vi "AscriptPluginMain.vi"(9 "StopNotifier":refnum<notifier>, 10 "IPnotifier":refnum<notifier>, 11 "BasePath":path) -> ()   [LabVIEW 2016]
uses:
  <vilib>/Utility/file.llb/Read Delimited Spreadsheet (string).vi
  <vilib>/Rock Robotics/Network Tables/NT Write Boolean.vi
  <vilib>/FTP/NI_FTP.lvlib
panel:
  out "RobotIP":string
  in  "DeleteLog":bool
  in  "GetLogFile":bool
  out "Auto Script on Robot":string="GotThroughDef3noShoot"
  in  "DLfromRIO":bool
  in  "TemplateOpen":bool
  in  "Autoscript Layout":string(tree)
  in  "DeleteCommand":bool
  in  "SaveStep":bool
  in  "DeleteStep":bool
  in  "AddCmd":bool
  in  "Auto Script Name":string="GotThroughDef3noShoot"
  in  "AutoFiles":i32(listbox)=7
  in  "LoadAuto":bool
  in  "SaveAuto":bool
  in  "ULtoRIO":bool
  in  "ClearSteps":bool
  in  "AddStep":bool
  in  "DeleteAuto":bool
  in  "Return Variable Names":string[](array[string])
  in  "Arguments":string[](array[string])
  in  "Routine":string(combo)
  in  "LoadStep":bool
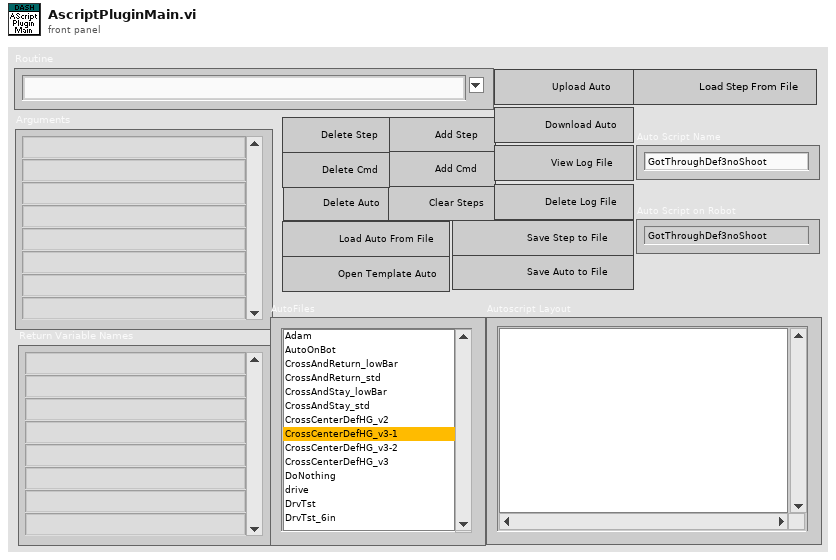
[diagram p1: front panel]
types:
  T1 = cluster{"Return Variable Names":refnum<vi>, "ArgumentsBox":refnum<vi>, "Routine":refnum<vi>, "AddCmd":refnum<vi>, "ClearSteps":refnum<vi>, "AddStep":refnum<vi>, "DeleteAuto":refnum<vi>, "DeleteCommand":refnum<vi>, "DeleteStep":refnum<vi>, "TemplateOpen":refnum<vi>, "SaveStep":refnum<vi>, "LoadAuto":refnum<vi>, "SaveAuto":refnum<vi>, "LoadStep":refnum<vi>, "AutoFiles":refnum<vi>, "DeleteLog":refnum<vi>, "GetLogFile":refnum<vi>, "Auto Script on Robot":refnum<vi>, "DLfromRIO":refnum<vi>, "Autoscript Layout":refnum<vi>, "Auto Script Name":refnum<vi>, "ULtoRIO":refnum<vi>}
  T2 = cluster{"Number":i32, "Name":string, "Commands":string[], "WaitForExecution":bool}
  T3 = enum16{"open", "replace", "create", "open or create", "replace or create", "replace or create with confirmation"}
  T4 = cluster{"Number":i32, "Name":string, "Commands":string[], "WaitForExecution":bool}[]
  T5 = typedef "NI_FTP.lvlib/FTP Session.ctl" = refnum<k5>
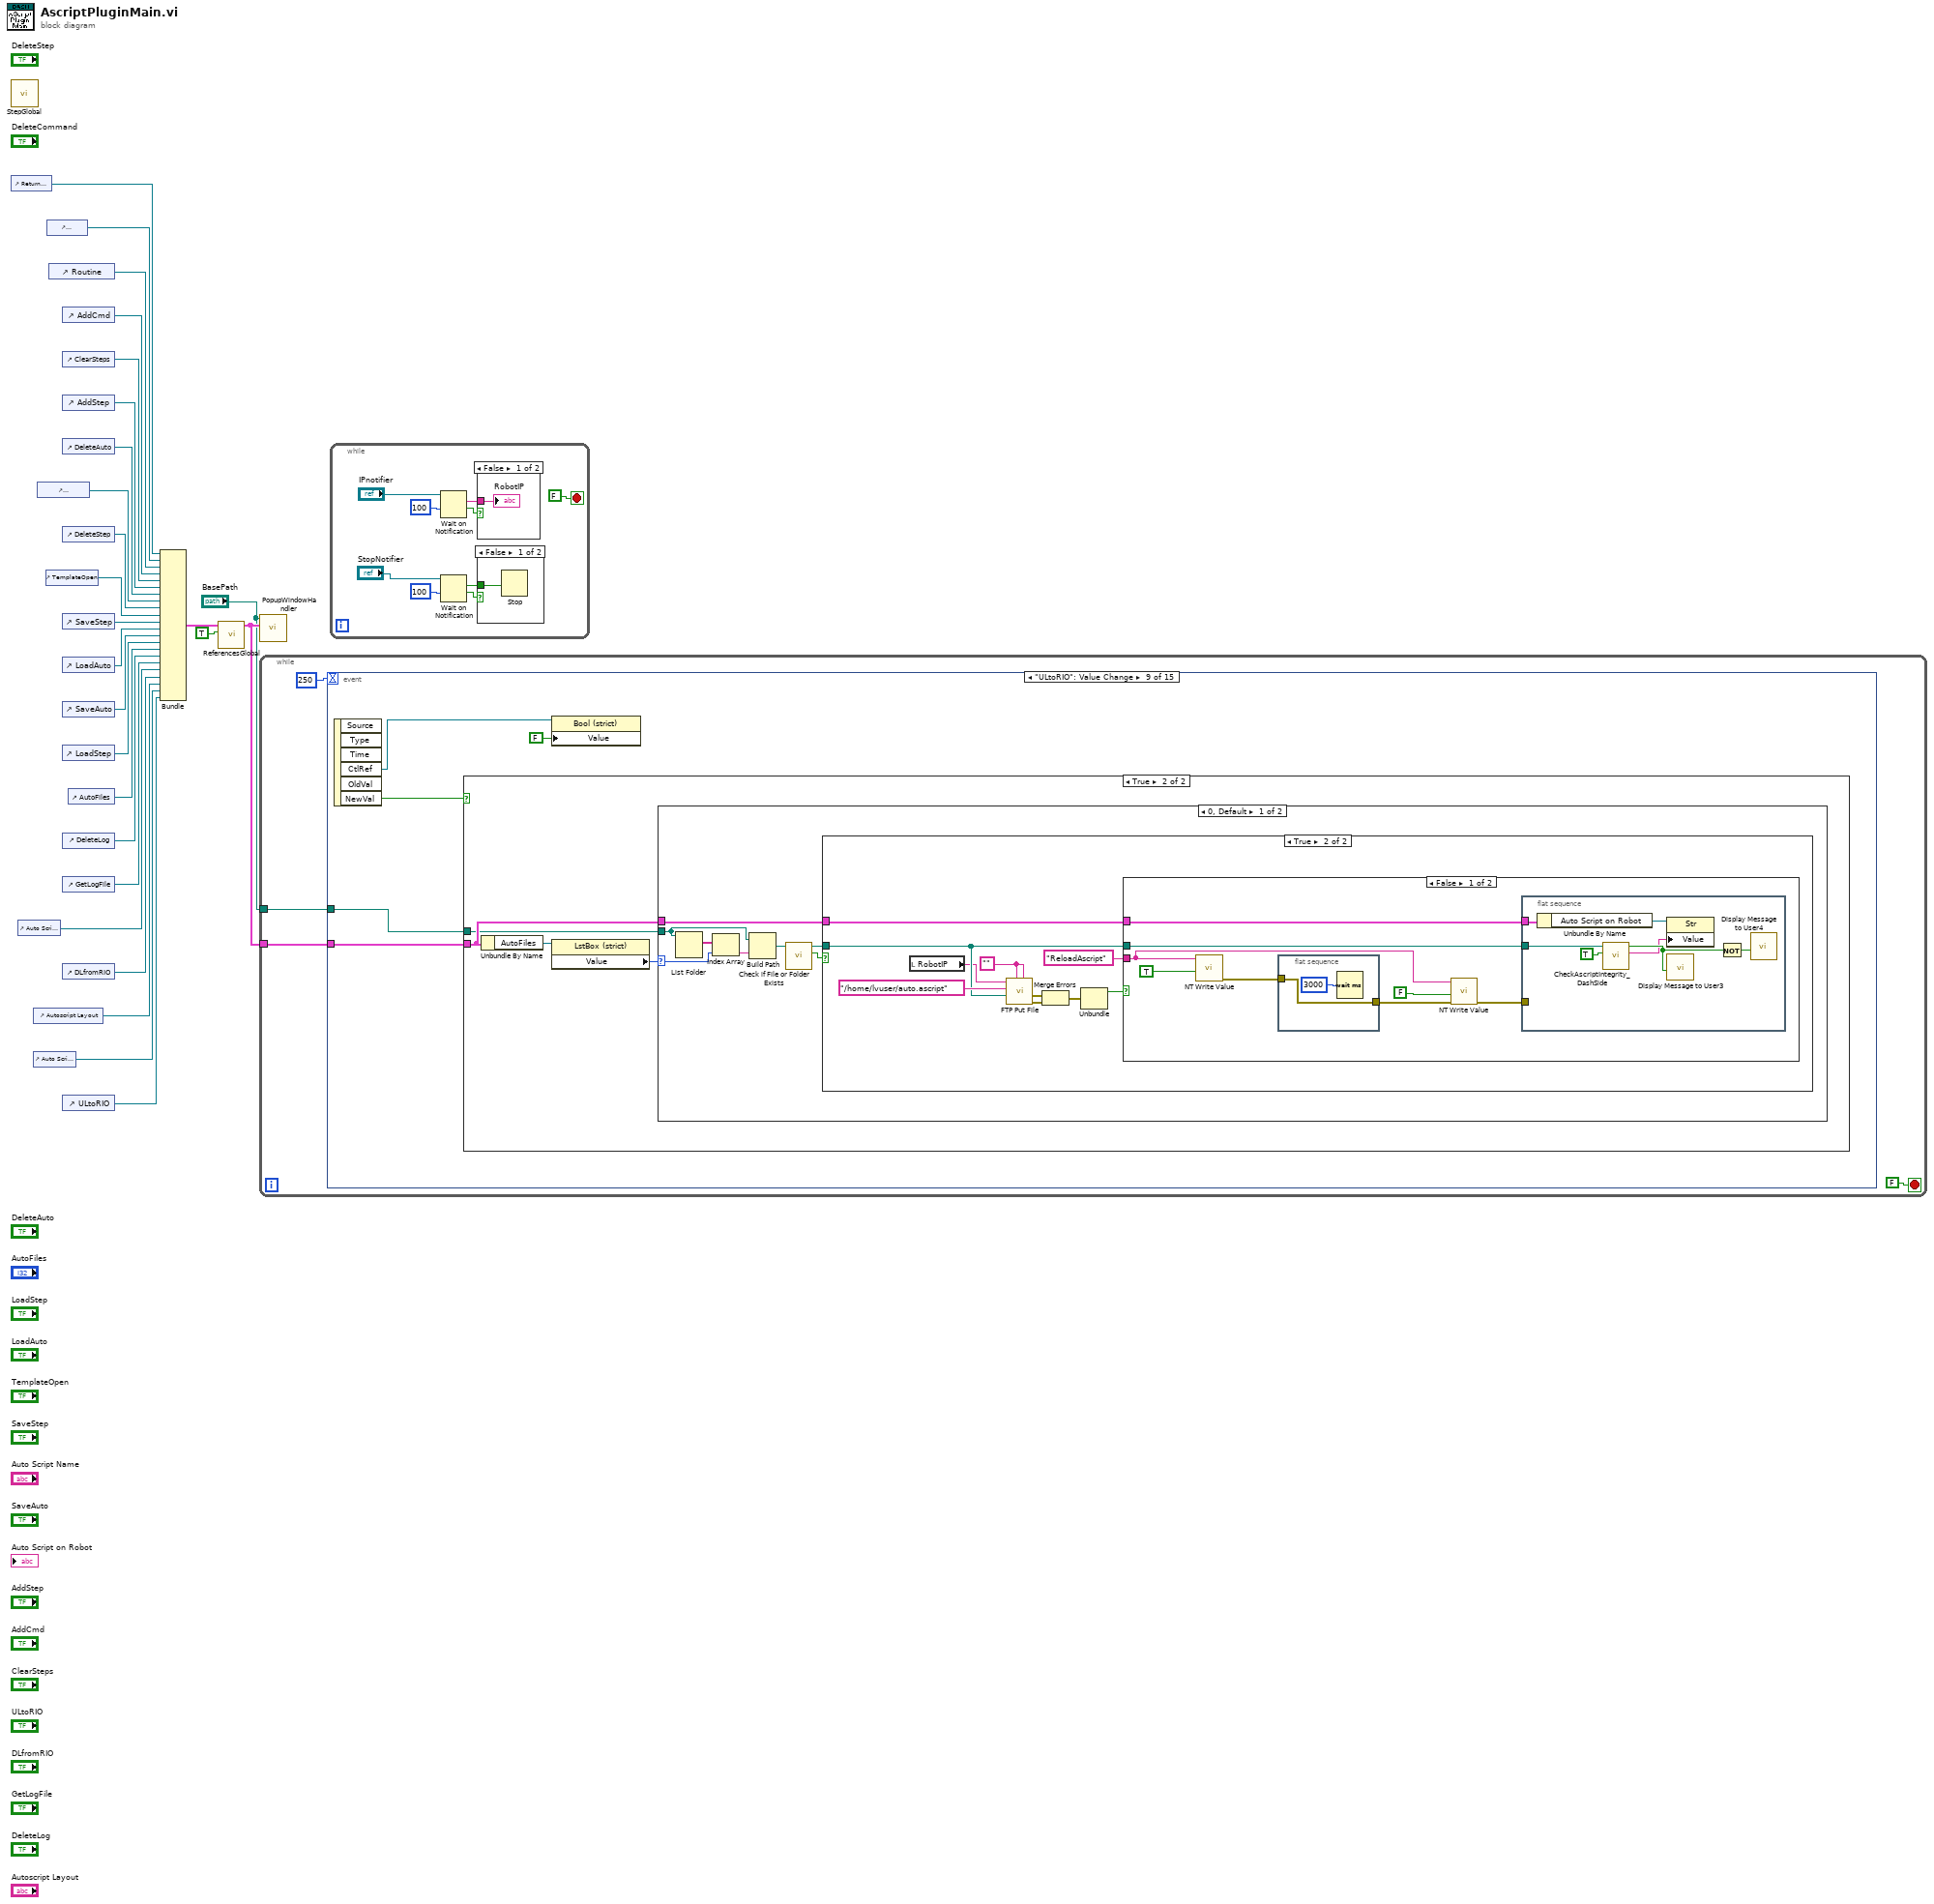
[diagram p0: block diagram]
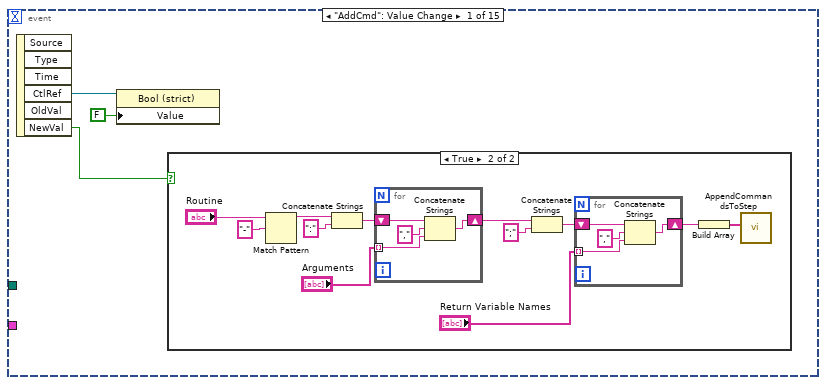
[diagram p2: hidden frame]
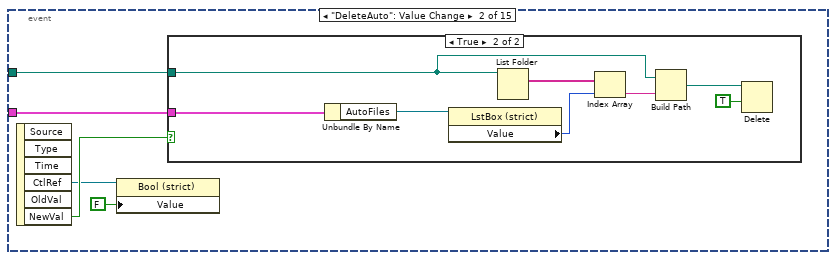
[diagram p4: hidden frame]
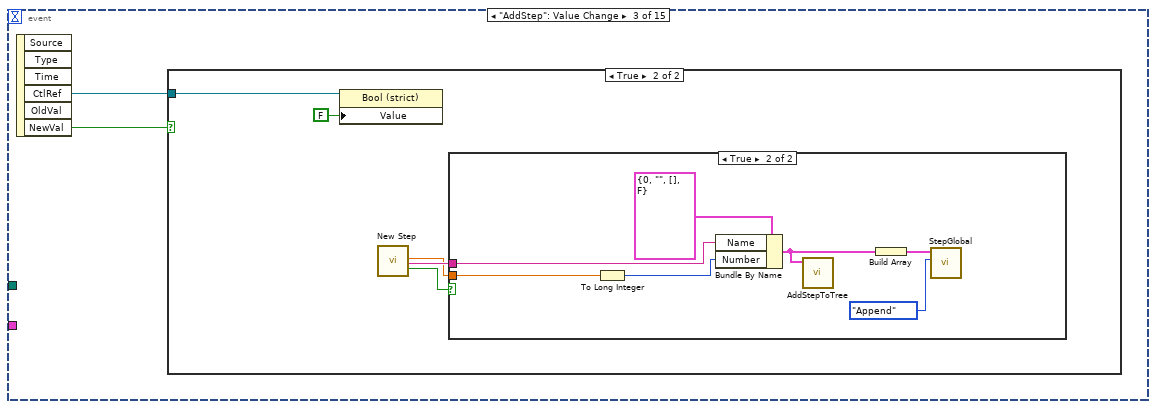
[diagram p6: hidden frame]
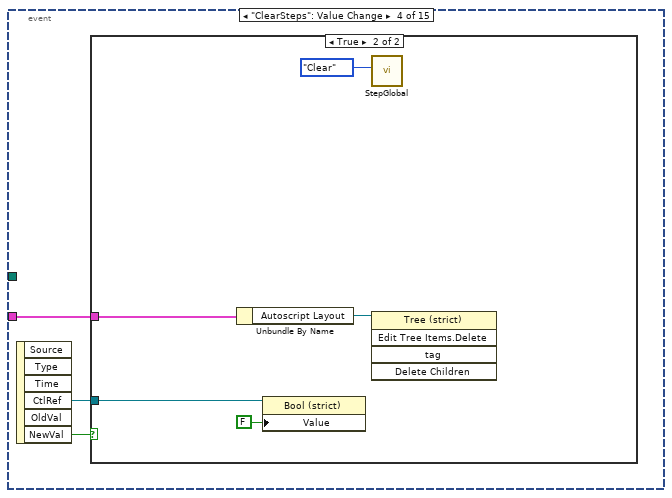
[diagram p9: hidden frame]
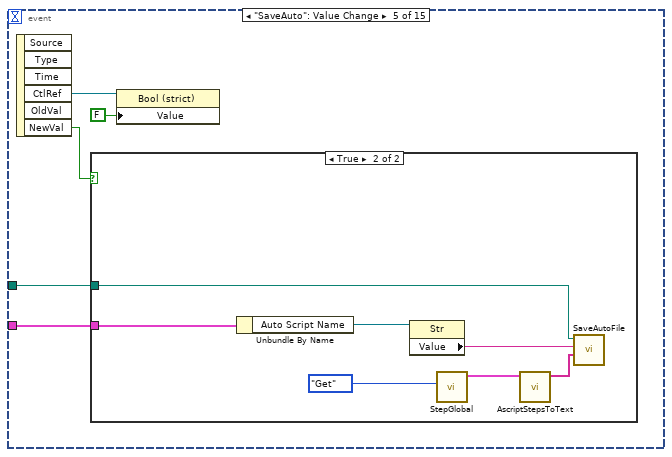
[diagram p11: hidden frame]
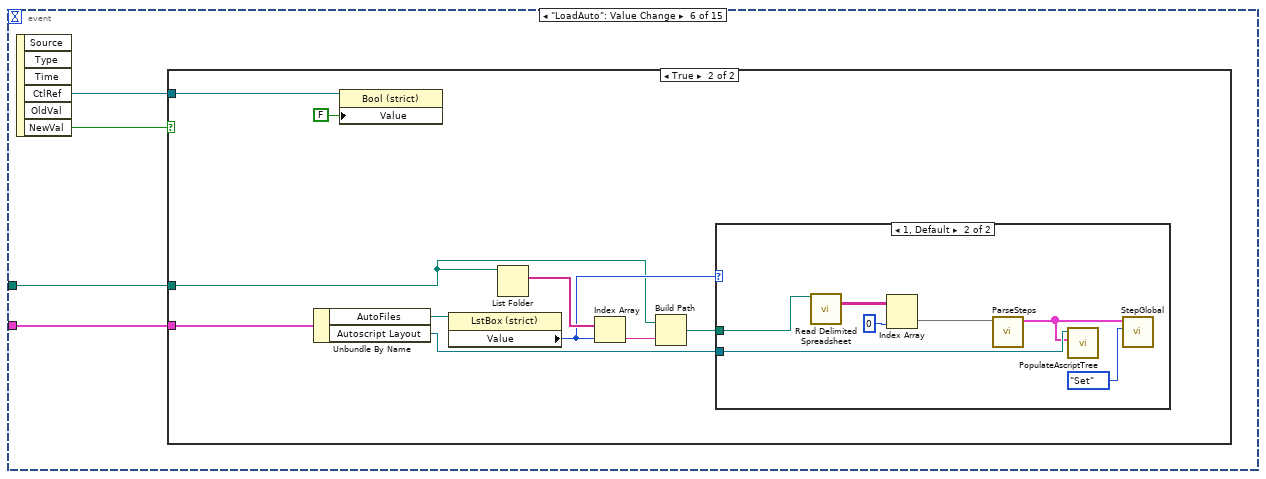
[diagram p13: hidden frame]
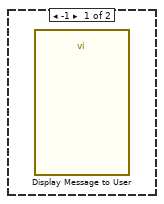
[diagram p15: hidden frame]
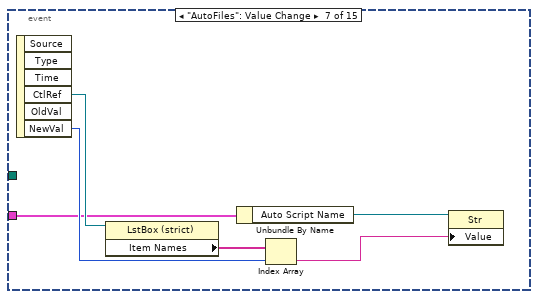
[diagram p16: hidden frame]
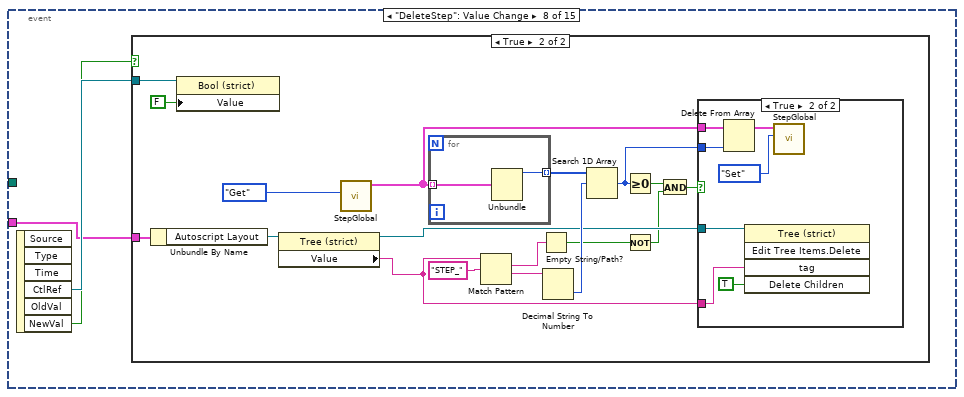
[diagram p17: hidden frame]
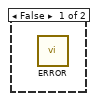
[diagram p19: hidden frame]
diagram:
  n1 = call "StepGlobal.vi"() -> ()  [unwired: 11 in, 1 out]
  n2 = control-ref of="Return Variable Names"() -> (w26:refnum<vi>)
  n3 = control-ref of="Auto Script on Robot"() -> (w9:refnum<vi>)
  n4 = control-ref of="Autoscript Layout"() -> (w7:refnum<vi>)
  n5 = control-ref of="Auto Script Name"() -> (w6:refnum<vi>)
  n6 = control-ref of="DeleteCommand"() -> (w19:refnum<vi>)
  n7 = control-ref of="TemplateOpen"() -> (w17:refnum<vi>)
  n8 = control-ref of="ArgumentsBox"() -> (w25:refnum<vi>)
  n9 = control-ref of="Routine"() -> (w24:refnum<vi>)
  n10 = control-ref of="AddCmd"() -> (w23:refnum<vi>)
  n11 = control-ref of="ClearSteps"() -> (w22:refnum<vi>)
  n12 = control-ref of="AddStep"() -> (w21:refnum<vi>)
  n13 = control-ref of="DeleteAuto"() -> (w20:refnum<vi>)
  n14 = control-ref of="DeleteStep"() -> (w18:refnum<vi>)
  n15 = control-ref of="SaveStep"() -> (w16:refnum<vi>)
  n16 = control-ref of="LoadAuto"() -> (w15:refnum<vi>)
  n17 = control-ref of="SaveAuto"() -> (w14:refnum<vi>)
  n18 = control-ref of="LoadStep"() -> (w13:refnum<vi>)
  n19 = control-ref of="DeleteLog"() -> (w10:refnum<vi>)
  n20 = control-ref of="GetLogFile"() -> (w11:refnum<vi>)
  n21 = control-ref of="DLfromRIO"() -> (w8:refnum<vi>)
  n22 = control-ref of="ULtoRIO"() -> (w5:refnum<vi>)
  n23 = control-ref of="AutoFiles"() -> (w12:refnum<vi>)
  n24 = Bundle("Return Variable Names"=w26, "ArgumentsBox"=w25, "Routine"=w24, "AddCmd"=w23, "ClearSteps"=w22, "AddStep"=w21, "DeleteAuto"=w20, "DeleteCommand"=w19, "DeleteStep"=w18, "TemplateOpen"=w17, "SaveStep"=w16, "LoadAuto"=w15, "SaveAuto"=w14, "LoadStep"=w13, "AutoFiles"=w12, "DeleteLog"=w10, "GetLogFile"=w11, "Auto Script on Robot"=w9, "DLfromRIO"=w8, "Autoscript Layout"=w7, "Auto Script Name"=w6, "ULtoRIO"=w5) -> (w4:T1)  [unwired: 1 in]
  n25 = call "ReferencesGlobal.vi"("Set?"=TRUE, "AscriptRefsIn"=w4) -> ("AscriptRefsOut"=w2:T1)  [unwired: 9 in]
  n26 = call "PopupWindowHandler.vi"("AscriptRefs"=w2, "BasePath"="BasePath") -> ()  [unwired: 10 in]
  n27 = while {
    tunnel: w2 -> [w30]
    tunnel: "BasePath" -> [w28]
    stop <- FALSE stop-if-true
    n28 = event shown="[8] \"ULtoRIO\": Value Change" {
      selector: _ -> [_ _ _ _ _ _ _ _ _ _ _ _ _ _ _]
      dyn-events: _ -> [_ _ _ _ _ _ _ _ _ _ _ _ _ _ _]
      timeout: 250 -> [_ _ _ _ _ _ _ _ _ _ _ _ _ _ _]
      tunnel: w30 -> [_ w58 _ w81 w93 w101 w122 w128 w162 _ w229 w262 _ _ w370]
      tunnel: w28 -> [_ w56 _ _ w92 w104 _ _ w161 w202 _ w258 w288 _ w369]
      event "AddCmd": Value Change {
        n29 = event-data() -> ("CtlRef"=w32:refnum<vi>, "NewVal"=w33:bool)  [unwired: 1 in, 4 out]
        n30 = property class="Bool (strict)"(reference=w32, "Value"=FALSE) -> ()  [unwired: 1 in, 2 out]
        n31 = case shown="True" w33 {
          frame False {
          }
          frame True {
            n32 = Match Pattern(string="Routine", regular expression="-") -> (before substring=w40:string)  [unwired: 1 in, 3 out]
            n33 = Concatenate Strings(w40, ":" ("string")) -> (w43:string)
            n34 = for {
              tunnel: "Arguments" -> [w52] mode=indexing
              shift-right: [w50] -> w35
              shift-left: w43 -> [w51]
              n35 = Concatenate Strings(w51, "," ("string"), w52) -> (w50:string)
            }
            n36 = Concatenate Strings(w35, ";" ("string")) -> (w37:string)
            n37 = for {
              tunnel: "Return Variable Names" -> [w48] mode=indexing
              shift-right: [w46] -> w34
              shift-left: w37 -> [w47]
              n38 = Concatenate Strings(w47, "," ("string"), w48) -> (w46:string)
            }
            n39 = Build Array(w34) -> (w45:string[])
            n40 = call "AppendCommandsToStep.vi"("CommandsToAppend"=w45) -> ()  [unwired: 11 in]
          }
        }
      }
      event "DeleteAuto": Value Change {
        n41 = event-data() -> ("CtlRef"=w54:refnum<vi>, "NewVal"=w57:bool)  [unwired: 1 in, 4 out]
        n42 = property class="Bool (strict)"(reference=w54, "Value"=FALSE) -> ()  [unwired: 1 in, 2 out]
        n43 = case shown="True" w57 {
          tunnel: w58 -> [_ w66]
          tunnel: w56 -> [_ w59]
          frame False {
          }
          frame True {
            n44 = Unbundle By Name(w66) -> ("AutoFiles"=w65:refnum<vi>)
            n45 = property class="LstBox (strict)"(reference=w65) -> ("Value"=w63:i32)  [unwired: 1 in, 2 out]
            n46 = List Folder(path=w59) -> (filenames=w64:string[])  [unwired: 3 in, 3 out]
            n47 = Index Array(array=w64, index=w63) -> (element=w62:string)
            n48 = Build Path(base path=w59, name or relative path=w62) -> (appended path=w60:path)
            n49 = Delete(path (use dialog)=w60, confirm (F)=TRUE) -> ()  [unwired: 3 in, 3 out]
          }
        }
      }
      event "AddStep": Value Change {
        n50 = event-data() -> ("CtlRef"=w68:refnum<vi>, "NewVal"=w67:bool)  [unwired: 1 in, 4 out]
        n51 = case shown="True" w67 {
          tunnel: w68 -> [_ w73]
          frame False {
          }
          frame True {
            n52 = property class="Bool (strict)"(reference=w73, "Value"=FALSE) -> ()  [unwired: 1 in, 2 out]
            n53 = call "New Step"() -> ("Step Number"=w69:dbl, "Step Name"=w70:string, "OK"=w71:bool)  [unwired: 16 in, 1 out]
            n54 = case shown="True" w71 {
              tunnel: w70 -> [_ w77]
              tunnel: w69 -> [_ w80]
              frame False {
              }
              frame True {
                n55 = To Long Integer(number=w80) -> (32bit integer=w78:i32)
                n56 = Bundle By Name(cluster=T2 {"Number"=0, "Name"="", "Commands"=[], "WaitForExecution"=FALSE} ("Step"), "Name"=w77, "Number"=w78) -> (w76:T2)
                n57 = call "AddStepToTree.vi"("Step"=w76) -> ()  [unwired: 10 in, 1 out]
                n58 = Build Array(w76) -> (w75:T4)
                n59 = call "StepGlobal.vi"("Action (Get)"=enum16{"Clear", "Append", "Set", "Get"}."Append" ("Action"), "AutoScriptSteps in"=w75) -> ()  [unwired: 9 in, 1 out]
              }
            }
          }
        }
      }
      event "ClearSteps": Value Change {
        n60 = event-data() -> ("CtlRef"=w83:refnum<vi>, "NewVal"=w82:bool)  [unwired: 1 in, 4 out]
        n61 = case shown="True" w82 {
          tunnel: w83 -> [_ w87]
          tunnel: w81 -> [_ w86]
          frame False {
          }
          frame True {
            n62 = Unbundle By Name(w86) -> ("Autoscript Layout"=w85:refnum<vi>)
            n63 = property class="Bool (strict)"(reference=w87, "Value"=FALSE) -> ()  [unwired: 1 in, 2 out]
            n64 = call "StepGlobal.vi"("Action (Get)"=enum16{"Clear", "Append", "Set", "Get"}."Clear" ("Action")) -> ()  [unwired: 10 in, 1 out]
            n65 = invoke class="Tree (strict)" method="Edit Tree Items.Delete"(reference=w85) -> ()  [unwired: 4 in, 5 out]
          }
        }
      }
      event "SaveAuto": Value Change {
        n66 = event-data() -> ("CtlRef"=w89:refnum<vi>, "NewVal"=w91:bool)  [unwired: 1 in, 4 out]
        n67 = case shown="True" w91 {
          tunnel: w93 -> [_ w100]
          tunnel: w92 -> [_ w94]
          frame False {
          }
          frame True {
            n68 = Unbundle By Name(w100) -> ("Auto Script Name"=w99:refnum<vi>)
            n69 = property class="Str"(reference=w99) -> ("Value"=w98:string)  [unwired: 1 in, 2 out]
            n70 = call "StepGlobal.vi"("Action (Get)"=enum16{"Clear", "Append", "Set", "Get"}."Get" ("Action")) -> ("AutoScriptSteps out"=w96:T4)  [unwired: 10 in]
            n71 = call "AscriptStepsToText.vi"("AutoScriptSteps"=w96) -> ("AscriptLines"=w97:string[])  [unwired: 10 in]
            n72 = call "SaveAutoFile.vi"("Ascript Data"=w97, "Filename"=w98, "Base path"=w94) -> ()  [unwired: 8 in, 1 out]
          }
        }
        n73 = property class="Bool (strict)"(reference=w89, "Value"=FALSE) -> ()  [unwired: 1 in, 2 out]
      }
      event "LoadAuto": Value Change {
        n74 = event-data() -> ("CtlRef"=w103:refnum<vi>, "NewVal"=w102:bool)  [unwired: 1 in, 4 out]
        n75 = case shown="True" w102 {
          tunnel: w101 -> [_ w110]
          tunnel: w103 -> [_ w109]
          tunnel: w104 -> [_ w105]
          frame False {
          }
          frame True {
            n76 = Unbundle By Name(w110) -> ("AutoFiles"=w113:refnum<vi>, "Autoscript Layout"=w106:refnum<vi>)
            n77 = property class="Bool (strict)"(reference=w109, "Value"=FALSE ("Panel Transparent")) -> ()  [unwired: 1 in, 2 out]
            n78 = property class="LstBox (strict)"(reference=w113) -> ("Value"=w108:i32)  [unwired: 1 in, 2 out]
            n79 = List Folder(path=w105) -> (filenames=w112:string[])  [unwired: 3 in, 3 out]
            n80 = Index Array(array=w112, index=w108) -> (element=w111:string)
            n81 = Build Path(base path=w105, name or relative path=w111) -> (appended path=w107:path)
            n82 = case shown="1, Default" w108 {
              tunnel: w107 -> [_ w121]
              tunnel: w106 -> [_ w117]
              frame -1 {
                n83 = call "Display Message to User"() -> ()  [unwired: 10 in, 2 out]
              }
              frame 1, Default {
                n84 = call-poly <vilib>:"Read Delimited Spreadsheet.vi"("file path (dialog if empty)"=w121) -> ("all rows"=w120:string[][])  [unwired: 9 in, 5 out]
                n85 = Index Array(array=w120, index (col)=0 ("disabled index (col)")) -> (element=w118:string[])  [unwired: 1 in]
                n86 = call "ParseSteps.vi"("AscriptLines"=w118) -> ("Steps"=w116:T4)  [unwired: 10 in]
                n87 = call "PopulateAscriptTree.vi"("Steps in"=w116, "Autoscript Layout"=w117) -> ()  [unwired: 8 in, 2 out]
                n88 = call "StepGlobal.vi"("Action (Get)"=enum16{"Clear", "Append", "Set", "Get"}."Set" ("Action"), "AutoScriptSteps in"=w116) -> ()  [unwired: 9 in, 1 out]
              }
            }
          }
        }
      }
      event "AutoFiles": Value Change {
        n89 = event-data() -> ("CtlRef"=w124:refnum<vi>, "NewVal"=w123:i32)  [unwired: 1 in, 4 out]
        n90 = property class="LstBox (strict)"(reference=w124) -> ("Item Names"=w125:string[])  [unwired: 1 in, 2 out]
        n91 = Unbundle By Name(w122) -> ("Auto Script Name"=w126:refnum<vi>)
        n92 = Index Array(array=w125, index=w123) -> (element=w127:string)
        n93 = property class="Str"(reference=w126, "Value"=w127) -> ()  [unwired: 1 in, 2 out]
      }
      event "DeleteStep": Value Change {
        n94 = event-data() -> ("CtlRef"=w130:refnum<vi>, "NewVal"=w129:bool)  [unwired: 1 in, 4 out]
        n95 = case shown="True" w129 {
          tunnel: w130 -> [_ w147]
          tunnel: w128 -> [_ w141]
          frame False {
          }
          frame True {
            n96 = Unbundle By Name(w141) -> ("Autoscript Layout"=w140:refnum<vi>)
            n97 = property class="Bool (strict)"(reference=w147, "Value"=FALSE ("Panel Transparent")) -> ()  [unwired: 1 in, 2 out]
            n98 = property class="Tree (strict)"(reference=w140) -> (reference out=w136:refnum<vi>, "Value"=w131:string)  [unwired: 1 in, 1 out]
            n99 = call "StepGlobal.vi"("Action (Get)"=enum16{"Clear", "Append", "Set", "Get"}."Get" ("Action")) -> ("AutoScriptSteps out"=w133:T4)  [unwired: 10 in]
            n100 = for {
              tunnel: w133 -> [w157] mode=indexing
              tunnel: [w156] -> w143 mode=indexing
              n101 = Unbundle(w157) -> ("Number"=w156:i32)  [unwired: 3 out]
            }
            n102 = Match Pattern(string=w131, regular expression="STEP_") -> (match substring=w137:string, after substring=w145:string)  [unwired: 1 in, 2 out]
            n103 = Empty String/Path?(string/path=w137) -> (empty?=w135:bool)
            n104 = Decimal String To Number(string=w145) -> (number=w144:i32)  [unwired: 2 in, 1 out]
            n105 = Search 1D Array(1D array=w143, element=w144) -> (index of element=w142:i32)  [unwired: 1 in]
            n106 = Greater Or Equal To 0?(x=w142) -> (x >= 0?=w139:bool)
            n107 = Not(x=w135) -> (.not. x?=w134:bool)
            n108 = And(x=w139, y=w134) -> (x .and. y?=w138:bool)
            n109 = case shown="True" w138 {
              tunnel: w142 -> [_ w155]
              tunnel: w133 -> [_ w154]
              tunnel: w136 -> [_ w153]
              tunnel: w131 -> [_ w152]
              frame False {
                n110 = call "ERROR"() -> ()  [unwired: 10 in, 2 out]
              }
              frame True {
                n111 = Delete From Array(array=w154, index=w155) -> (array with subset deleted=w150:T4)  [unwired: 1 in, 1 out]
                n112 = invoke class="Tree (strict)" method="Edit Tree Items.Delete"(reference=w153, "tag"=w152, "Delete Children"=TRUE ("Delete Children?")) -> ()  [unwired: 2 in, 5 out]
                n113 = call "StepGlobal.vi"("Action (Get)"=enum16{"Clear", "Append", "Set", "Get"}."Set" ("Action"), "AutoScriptSteps in"=w150) -> ()  [unwired: 9 in, 1 out]
              }
            }
          }
        }
      }
      event "ULtoRIO": Value Change {
        n114 = event-data() -> ("CtlRef"=w158:refnum<vi>, "NewVal"=w160:bool)  [unwired: 1 in, 4 out]
        n115 = case shown="True" w160 {
          tunnel: w162 -> [_ w164]
          tunnel: w161 -> [_ w163]
          frame False {
          }
          frame True {
            n116 = Unbundle By Name(w164) -> ("AutoFiles"=w166:refnum<vi>)
            n117 = property class="LstBox (strict)"(reference=w166) -> ("Value"=w165:i32)  [unwired: 1 in, 2 out]
            n118 = case shown="0, Default" w165 {
              selector: w165 -> [w172 _]
              tunnel: w164 -> [w168 _]
              tunnel: w163 -> [w167 _]
              frame 0, Default {
                n119 = List Folder(path=w167) -> (filenames=w174:string[])  [unwired: 3 in, 3 out]
                n120 = Index Array(array=w174, index=w172) -> (element=w173:string)
                n121 = Build Path(base path=w167, name or relative path=w173) -> (appended path=w171:path)
                n122 = call <vilib>:"Check if File or Folder Exists.vi"("path"=w171) -> ("file or folder exists?"=w170:bool, "dup path"=w169:path)  [unwired: 8 in, 1 out]
                n123 = case shown="True" w170 {
                  tunnel: w169 -> [_ w177]
                  tunnel: w168 -> [_ w176]
                  frame False {
                    n124 = call "Display Message to User2"() -> ()  [unwired: 10 in, 2 out]
                  }
                  frame True {
                    w180 = ""
                    n125 = local read "RobotIP"() -> (w175:string)
                    n126 = call <vilib>:"FTP Put File.vi"("password"=w180, "user"=w180, "local path"=w177, "remote path"="/home/lvuser/auto.ascript" ("remote path (roboRIO)"), "host"=w175) -> ("error out"=w183:errorcluster, "file error"=w184:errorcluster)  [unwired: 5 in]
                    n127 = Merge Errors(w184, w183) -> (w182:errorcluster)
                    n128 = Unbundle(w182) -> ("status"=w179:bool)  [unwired: 2 out]
                    n129 = case shown="False" w179 {
                      tunnel: "ReloadAscript" ("remote path (roboRIO)") -> [w189 _]
                      tunnel: w177 -> [w186 _]
                      tunnel: w176 -> [w185 _]
                      frame False {
                        n130 = call-poly <vilib>:"NT Write Value.vi"("Boolean"=TRUE, "Name"=w189) -> ("error out"=w191:errorcluster)  [unwired: 9 in]
                        n131 = flat-sequence {
                          tunnel: w191 -> [w200]
                          tunnel: [w200] -> w190
                          frame #0 {
                            n132 = Wait (ms)(milliseconds to wait=u32 3000) -> ()  [unwired: 1 out]
                          }
                        }
                        n133 = call-poly <vilib>:"NT Write Value.vi"("error in"=w190, "Boolean"=FALSE, "Name"=w189) -> ("error out"=w187:errorcluster)  [unwired: 8 in]
                        n134 = flat-sequence {
                          tunnel: w187 -> [_]
                          tunnel: w186 -> [w198]
                          tunnel: w185 -> [w195]
                          frame #0 {
                            n135 = Unbundle By Name(w195) -> ("Auto Script on Robot"=w194:refnum<vi>)
                            n136 = call "CheckAscriptIntegrity_DashSide.vi"("UseUploadedPath?"=TRUE, "UploadedAscript"=w198) -> ("BotAscriptName"=w193:string, "AscriptIntegrityGood?"=w196:bool)  [unwired: 8 in]
                            n137 = property class="Str"(reference=w194, "Value"=w193) -> ()  [unwired: 1 in, 2 out]
                            n138 = call "Display Message to User3"("Enable"=w196) -> ()  [unwired: 9 in, 2 out]
                            n139 = Not(x=w196) -> (.not. x?=w197:bool)
                            n140 = call "Display Message to User4"("Enable"=w197) -> ()  [unwired: 9 in, 2 out]
                          }
                        }
                      }
                      frame True {
                        n141 = call "Display Message to User5"() -> ()  [unwired: 10 in, 2 out]
                      }
                    }
                  }
                }
              }
              frame -1 {
                n142 = call "Display Message to User6"() -> ()  [unwired: 10 in, 2 out]
              }
            }
          }
        }
        n143 = property class="Bool (strict)"(reference=w158, "Value"=FALSE ("Panel Transparent")) -> ()  [unwired: 1 in, 2 out]
      }
      event "SaveStep": Value Change {
        n144 = event-data() -> ("CtlRef"=w203:refnum<vi>, "NewVal"=w204:bool)  [unwired: 1 in, 4 out]
        n145 = case shown="True" w204 {
          tunnel: w203 -> [_ w206]
          tunnel: w202 -> [_ w205]
          frame False {
          }
          frame True {
            n146 = property class="Bool (strict)"(reference=w206, "Value"=FALSE) -> ()  [unwired: 1 in, 2 out]
            n147 = call "Save Step"() -> ("Step Name"=w207:string, "Use Existing Step Name?"=w208:bool, "Step Number"=w210:dbl, "OK"=w211:bool)  [unwired: 15 in, 1 out]
            n148 = To Long Integer(number=w210) -> (32bit integer=w209:i32)
            n149 = case shown="True" w211 {
              tunnel: w209 -> [_ w220]
              tunnel: w208 -> [_ w218]
              tunnel: w207 -> [_ w216]
              tunnel: w205 -> [_ w213]
              frame False {
              }
              frame True {
                n150 = call "StepGlobal.vi"() -> ("AutoScriptSteps out"=w214:T4)  [unwired: 11 in]
                n151 = for {
                  tunnel: w214 -> [w227] mode=indexing
                  tunnel: [w226] -> w221 mode=indexing
                  n152 = Unbundle(w227) -> ("Number"=w226:i32)  [unwired: 3 out]
                }
                n153 = Search 1D Array(1D array=w221, element=w220) -> (index of element=w219:i32)  [unwired: 1 in]
                n154 = Index Array(array=w214, index=w219) -> (element=w217:T2)
                n155 = case shown="True" w218 {
                  tunnel: w217 -> [w224 w225]
                  tunnel: w216 -> [w223 _]
                  tunnel: [w222 w225] -> w215
                  frame False {
                    n156 = Bundle By Name(cluster=w224, "Name"=w223) -> (w222:T2)
                  }
                  frame True {
                  }
                }
                n157 = call "SaveStepToFile.vi"("base path"=w213, "Step"=w215) -> ()  [unwired: 10 in]
              }
            }
          }
        }
      }
      event "DeleteCommand": Value Change {
        n158 = event-data() -> ("CtlRef"=w230:refnum<vi>, "NewVal"=w228:bool)  [unwired: 1 in, 4 out]
        n159 = property class="Bool (strict)"(reference=w230, "Value"=FALSE) -> ()  [unwired: 1 in, 2 out]
        n160 = case shown="True" w228 {
          tunnel: w229 -> [_ w236]
          frame False {
          }
          frame True {
            n161 = Unbundle By Name(w236) -> ("Autoscript Layout"=w235:refnum<vi>)
            n162 = property class="Tree (strict)"(reference=w235) -> (reference out=w233:refnum<vi>, "Value"=w232:string)  [unwired: 1 in, 1 out]
            n163 = Empty String/Path?(string/path=w232) -> (empty?=w234:bool)
            n164 = case shown="False" w234 {
              tunnel: w232 -> [w241 _]
              tunnel: w233 -> [w240 _]
              frame False {
                n165 = invoke class="Tree (strict)" method="Edit Tree Items.Delete"(reference=w240, "tag"=w241, "Delete Children"=TRUE ("Delete Children?")) -> ()  [unwired: 2 in, 5 out]
                n166 = call "StepGlobal.vi"() -> ("AutoScriptSteps out"=w239:T4)  [unwired: 11 in]
                n167 = Match Pattern(string=w241, regular expression="_") -> (before substring=w245:string, after substring=w246:string)  [unwired: 1 in, 2 out]
                n168 = for {
                  tunnel: w239 -> [w257] mode=indexing
                  tunnel: [w256] -> w249 mode=indexing
                  n169 = Unbundle By Name(w257) -> ("Number"=w256:i32)
                }
                n170 = Decimal String To Number(string=w245) -> (number=w244:i32)  [unwired: 2 in, 1 out]
                n171 = Decimal String To Number(string=w246) -> (number=w243:i32)  [unwired: 2 in, 1 out]
                n172 = Search 1D Array(1D array=w249, element=w244) -> (index of element=w248:i32)  [unwired: 1 in]
                n173 = in-place {
                  in-place-border: w243 -> [w251]
                  n174 = in-place-array #1(w239, w248) -> (w252:T2)
                  n175 = in-place {
                    in-place-border: w251 -> [w253]
                    n176 = in-place-cluster #2(w252) -> ("Commands"=w255:string[])
                    n177 = Delete From Array(array=w255, index=w253) -> (array with subset deleted=w254:string[])  [unwired: 1 in, 1 out]
                    n178 = in-place-cluster #2("Commands"=w254) -> (w250:T2)
                  }
                  n179 = in-place-array #1(w250) -> (w238:T4)  [unwired: 1 out]
                }
                n180 = call "StepGlobal.vi"("Action (Get)"=enum16{"Clear", "Append", "Set", "Get"}."Set", "AutoScriptSteps in"=w238) -> ()  [unwired: 9 in, 1 out]
              }
              frame True {
              }
            }
          }
        }
      }
      event "DLfromRIO": Value Change {
        n181 = event-data() -> ("CtlRef"=w259:refnum<vi>, "NewVal"=w261:bool)  [unwired: 1 in, 4 out]
        n182 = property class="Bool (strict)"(reference=w259, "Value"=FALSE) -> ()  [unwired: 1 in, 2 out]
        n183 = case shown="True" w261 {
          tunnel: w262 -> [_ w266]
          tunnel: w258 -> [_ w264]
          frame False {
          }
          frame True {
            w275 = ""
            n184 = call <vilib>:"Check if File or Folder Exists.vi"("path"=w264) -> ("file or folder exists?"=w277:bool, "dup path"=w276:path)  [unwired: 8 in, 1 out]
            n185 = case shown="False" w277 {
              tunnel: w276 -> [w286 w287]
              tunnel: [w285 w287] -> w273
              frame False {
                n186 = Create Folder(path (use dialog)=w286) -> (created path=w285:path)  [unwired: 2 in, 2 out]
              }
              frame True {
              }
            }
            n187 = local read "RobotIP"() -> (w263:string)
            n188 = Build Path(base path=w273, name or relative path="AutoOnBot.ascript") -> (appended path=w267:path)
            n189 = call <vilib>:"FTP Get File.vi"("password"=w275, "user"=w275, "local path"=w267, "remote path"="/home/lvuser/auto.ascript", "host"=w263) -> ("error out"=w270:errorcluster, "file error"=w271:errorcluster)  [unwired: 5 in]
            n190 = Unbundle By Name(w266) -> ("Autoscript Layout"=w265:refnum<vi>)
            n191 = Merge Errors(w271, w270) -> (w269:errorcluster)
            n192 = Unbundle(w269) -> ("status"=w268:bool)  [unwired: 2 out]
            n193 = case shown="False" w268 {
              tunnel: w267 -> [w281 _]
              tunnel: w265 -> [w280 _]
              frame False {
                n194 = call-poly <vilib>:"Read Delimited Spreadsheet.vi"("file path (dialog if empty)"=w281) -> ("all rows"=w284:string[][])  [unwired: 9 in, 5 out]
                n195 = Index Array(array=w284, index (col)=0 ("disabled index (col)")) -> (element=w282:string[])  [unwired: 1 in]
                n196 = call "ParseSteps.vi"("AscriptLines"=w282) -> ("Steps"=w279:T4)  [unwired: 10 in]
                n197 = call "PopulateAscriptTree.vi"("Steps in"=w279, "Autoscript Layout"=w280) -> ()  [unwired: 8 in, 2 out]
                n198 = call "StepGlobal.vi"("Action (Get)"=enum16{"Clear", "Append", "Set", "Get"}."Set", "AutoScriptSteps in"=w279) -> ()  [unwired: 9 in, 1 out]
              }
              frame True {
                n199 = call "Display Message to User7"() -> ()  [unwired: 10 in, 2 out]
              }
            }
          }
        }
      }
      event "GetLogFile": Value Change {
        n200 = event-data() -> ("CtlRef"=w289:refnum<vi>, "NewVal"=w290:bool)  [unwired: 1 in, 4 out]
        n201 = property class="Bool (strict)"(reference=w289, "Value"=FALSE) -> ()  [unwired: 1 in, 2 out]
        n202 = case shown="True" w290 {
          tunnel: w288 -> [_ w293]
          frame False {
          }
          frame True {
            w304 = ""
            n203 = Build Path(base path=w293, name or relative path="AutoLogFiles") -> (appended path=w307:path)
            n204 = call <vilib>:"Check if File or Folder Exists.vi"("path"=w307) -> ("file or folder exists?"=w306:bool, "dup path"=w305:path)  [unwired: 8 in, 1 out]
            n205 = case shown="False" w306 {
              tunnel: w305 -> [w316 w317]
              tunnel: [w315 w317] -> w302
              frame False {
                n206 = Create Folder(path (use dialog)=w316) -> (created path=w315:path)  [unwired: 2 in, 2 out]
              }
              frame True {
              }
            }
            n207 = Get Date/Time In Seconds() -> (seconds since 1Jan1904=w298:timestamp)
            n208 = Format Date/Time String(time format string (%c)="AutoLog__%m-%d-%y_%H-%M.txt", seconds (now)=w298) -> (date/time string=w296:string)  [unwired: 1 in]
            n209 = Build Path(base path=w302, name or relative path=w296) -> (appended path=w294:path)
            n210 = local read "RobotIP"() -> (w292:string)
            n211 = call <vilib>:"FTP Get File.vi"("password"=w304, "user"=w304, "local path"=w294, "remote path"="/home/lvuser/AutoLog.txt", "host"=w292) -> ("error out"=w300:errorcluster, "file error"=w301:errorcluster)  [unwired: 5 in]
            n212 = Merge Errors(w301, w300) -> (w299:errorcluster)
            n213 = Unbundle(w299) -> ("status"=w295:bool)  [unwired: 2 out]
            n214 = case shown="False" w295 {
              tunnel: w294 -> [w310 _]
              frame False {
                n215 = Strip Path(path=w310) -> (stripped path=w314:path, name=w312:string)
                n216 = Concatenate Strings("notepad " ("string"), w312) -> (w311:string)
                n217 = call <vilib>:"System Exec.vi"("wait until completion? (T)"=FALSE, "working directory"=w314, "command line"=w311) -> ()  [unwired: 5 in, 4 out]
              }
              frame True {
                n218 = call "Display Message to User8"() -> ()  [unwired: 10 in, 2 out]
              }
            }
          }
        }
      }
      event "DeleteLog": Value Change {
        n219 = event-data() -> ("CtlRef"=w318:refnum<vi>, "NewVal"=w319:bool)  [unwired: 1 in, 4 out]
        n220 = property class="Bool (strict)"(reference=w318, "Value"=FALSE) -> (error out=w321:errorcluster)  [unwired: 1 in, 1 out]
        n221 = case shown="True" w319 {
          tunnel: w321 -> [_ _]
          frame False {
          }
          frame True {
            n222 = call "Display Message to User9"() -> ("OK"=w322:bool)  [unwired: 10 in, 1 out]
            n223 = case shown="True" w322 {
              frame False {
              }
              frame True {
                w347 = ""
                n224 = local read "RobotIP"() -> (w323:string)
                n225 = call <vilib>:"FTP Open Session.vi"("timeout ms (60000)"=10000, "address"=w323) -> ("error out"=w344:errorcluster, "reply string"=w341:string, "reply code"=w342:i32, "ftp session"=w343:T5)  [unwired: 6 in]
                n226 = call <vilib>:"FTP Reply To Error.vi"("error in (no error)"=w344, "reply string in"=w341, "reply code in"=w342, "ftp session"=w343) -> ("error out"=w339:errorcluster, "ftp session out"=w340:T5)  [unwired: 2 out]
                n227 = call <vilib>:"FTP Logon.vi"("starting path"="/home/lvuser", "error in (no error)"=w339, "password"=w347, "user"=w347, "ftp session"=w340) -> ("error out"=w336:errorcluster, "reply string"=w335:string, "reply code"=w334:i32, "ftp session out"=w337:T5)  [unwired: 3 in]
                n228 = call <vilib>:"FTP Reply To Error.vi"("error in (no error)"=w336, "reply string in"=w335, "reply code in"=w334, "ftp session"=w337) -> ("error out"=w338:errorcluster, "ftp session out"=w333:T5)  [unwired: 2 out]
                n229 = call <vilib>:"FTP Command.vi"("error in (no error)"=w338, "command"="delete AutoLog.txt", "ftp session"=w333) -> ("error out"=w331:errorcluster, "reply string"=w330:string, "reply code"=w329:i32, "ftp session out"=w332:T5)  [unwired: 5 in]
                n230 = call <vilib>:"FTP Reply To Error.vi"("error in (no error)"=w331, "reply string in"=w330, "reply code in"=w329, "ftp session"=w332) -> ("error out"=w327:errorcluster, "ftp session out"=w328:T5)  [unwired: 2 out]
                n231 = call <vilib>:"FTP Close Session.vi"("error in (no error)"=w327, "ftp session"=w328) -> ("error out"=w326:errorcluster)  [unwired: 6 in, 3 out]
                n232 = case shown="Error" w326 {
                  selector: w326 -> [_ w355]
                  tunnel: "Failed to delete log file. Details:\n\n" -> [_ w351]
                  tunnel: ["Successfully deleted Auto log file." ("f") w350] -> w324
                  frame No Error {
                  }
                  frame Error {
                    n233 = Unbundle By Name(w355) -> ("code"=w353:i32, "source"=w352:string)
                    n234 = Format Into String(format string="Error %d: %s", initial string=w351, w353, w352) -> (resulting string=w350:string)  [unwired: 1 in, 1 out]
                  }
                }
                n235 = call "Display Message to User10"("Message"=w324) -> ()  [unwired: 9 in, 2 out]
              }
            }
          }
        }
      }
      event Timeout {
        n236 = event-data() -> ()  [unwired: 1 in, 3 out]
        n237 = call <vilib>:"Check if File or Folder Exists.vi"("path"=w369) -> ("file or folder exists?"=w371:bool, "dup path"=w372:path)  [unwired: 8 in, 1 out]
        n238 = case shown="True" w371 {
          tunnel: w372 -> [w395 w396]
          tunnel: [w394 w396] -> w373
          frame False {
            n239 = Create Folder(path (use dialog)=w395) -> (created path=w394:path)  [unwired: 2 in, 2 out]
          }
          frame True {
          }
        }
        n240 = List Folder(path=w373) -> (path out=w368:path, filenames=w375:string[])  [unwired: 3 in, 2 out]
        n241 = Build Path(base path=w368, name or relative path="Config") -> (appended path=w364:path)
        n242 = for {
          tunnel: w368 -> [w393]
          tunnel: w375 -> [w392] mode=indexing
          tunnel: [w390] -> w376 mode=indexing
          n243 = Build Path(base path=w393, name or relative path=w392) -> (appended path=w391:path)
          n244 = call <vilib>:"Get File Extension.vi"("file"=w391) -> ("filename without extension"=w390:string)  [unwired: 6 in, 4 out]
        }
        n245 = call <vilib>:"Check if File or Folder Exists.vi"("path"=w364) -> ("file or folder exists?"=w366:bool, "dup path"=w365:path)  [unwired: 8 in, 1 out]
        n246 = case shown="False" w366 {
          tunnel: w365 -> [w388 w389]
          tunnel: [w387 w389] -> w363
          frame False {
            n247 = Create Folder(path (use dialog)=w388) -> (created path=w387:path)  [unwired: 2 in, 2 out]
          }
          frame True {
          }
        }
        n248 = Build Path(base path=w363, name or relative path="AutoScriptCommands.txt") -> (appended path=w360:path)
        n249 = call <vilib>:"Check if File or Folder Exists.vi"("path"=w360) -> ("file or folder exists?"=w359:bool, "dup path"=w358:path)  [unwired: 8 in, 1 out]
        n250 = case shown="False" w359 {
          tunnel: w358 -> [w382 w386]
          tunnel: [_ w383] -> w357
          frame False {
            n251 = Open/Create/Replace File(file path (use dialog)=w382, operation (0:open)=T3."create") -> (refnum out=w379:refnum<file>, error out=w380:errorcluster)  [unwired: 4 in, 1 out]
            n252 = Close File(refnum=w379, error in=w380) -> ()  [unwired: 2 out]
          }
          frame True {
            n253 = call-poly <vilib>:"Read Delimited Spreadsheet.vi"("file path (dialog if empty)"=w386) -> ("all rows"=w384:string[][])  [unwired: 9 in, 5 out]
            n254 = Index Array(array=w384, index (col)=0 ("disabled index (col)")) -> (element=w383:string[])  [unwired: 1 in]
          }
        }
        n255 = Unbundle By Name(w370) -> ("Routine"=w361:refnum<vi>, "Auto Script on Robot"=w377:refnum<vi>, "AutoFiles"=w374:refnum<vi>)
        n256 = Build Cluster Array(w357, w357) -> (w356:cluster{"String":string, "String":string}[])
        n257 = call "CheckAscriptIntegrity_DashSide.vi"() -> ("BotAscriptName"=w378:string)  [unwired: 10 in, 1 out]
        n258 = property class="CmbBox"(reference=w361, "Strings And Values[]"=w356) -> ()  [unwired: 1 in, 2 out]
        n259 = property class="Str"(reference=w377, "Value"=w378) -> ()  [unwired: 1 in, 2 out]
        n260 = property class="LstBox (strict)"(reference=w374, "Item Names"=w376) -> ()  [unwired: 1 in, 2 out]
      }
    }
  }
  n261 = while {
    stop <- FALSE stop-if-true
    n262 = Wait on Notification(notifier="IPnotifier", timeout in ms (-1)=100) -> (notification=w403:string, timed out?=w404:bool)  [unwired: 2 in, 2 out]
    n263 = Wait on Notification(notifier="StopNotifier", timeout in ms (-1)=100) -> (notification=w399:bool, timed out?=w398:bool)  [unwired: 2 in, 2 out]
    n264 = case shown="False" w404 {
      tunnel: w403 -> [w407 _]
      frame False {
        "RobotIP" <- w407
      }
      frame True {
      }
    }
    n265 = case shown="False" w398 {
      tunnel: w399 -> [w406 _]
      frame False {
        n266 = Stop(stop? (T)=w406) -> ()
      }
      frame True {
      }
    }
  }
